vi "mpu.vi"() -> ()   [LabVIEW 2019]
panel:
  out "error out":errorcluster
  in  "error in":errorcluster {"code" format="%.0x"}
  in  "?":i32(slide)=7 scale=20.0..50.0
  in  "Вкл.":bool
  out "Крен, град":dbl(graph)
  out "Тангаж":cluster{i32, dbl}(graph)
  out "?":dbl
  out "Крен, град":dbl(knob) scale=-180.0..180.0
  out "?":dbl
  out "Тангаж, град.":dbl(knob) scale=-180.0..180.0
  in  "Порт:":refnum<visa-resource-name>
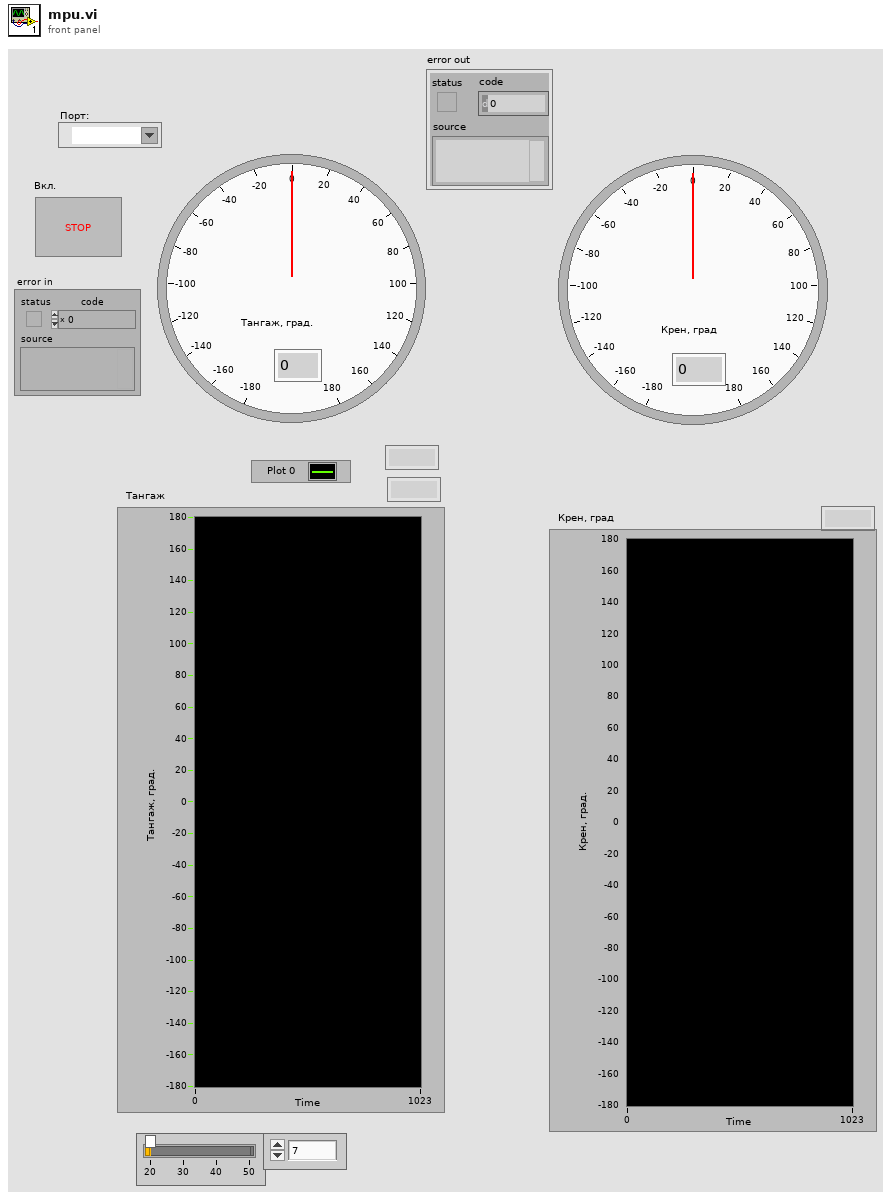
[diagram p1: front panel]
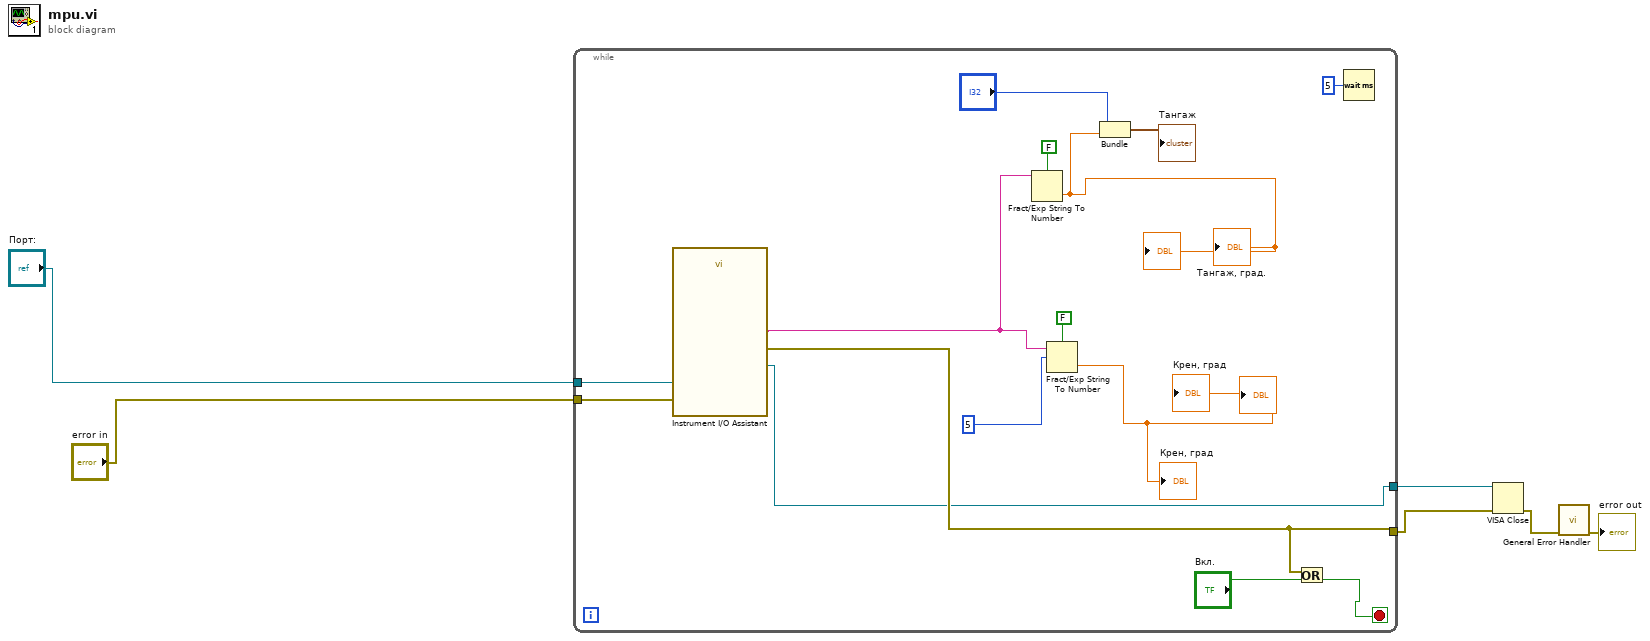
[diagram p0: block diagram]
diagram:
  n1 = while {
    tunnel: [w8] -> w6
    tunnel: "Порт:" -> [w11]
    tunnel: "error in" -> [w10]
    tunnel: [w7] -> w1
    stop <- w12 stop-if-true
    n2 = call "Instrument I/O Assistant"("Session In"=w11, "error in"=w10) -> ("Session Out"=w7:refnum<visa-resource-name>, "token"=w9:string, "error out"=w8:errorcluster)  [unwired: 23 in]
    n3 = Fract/Exp String To Number(use system decimal point (T)=FALSE, string=w9) -> (number=w16:dbl)  [unwired: 2 in, 1 out]
    "Тангаж, град." <- w16
    "?" <- w16
    n4 = Fract/Exp String To Number(use system decimal point (T)=FALSE, string=w9, offset=5) -> (number=→"Крен, град" →"?" →"Крен, град":dbl)  [unwired: 1 in, 1 out]
    n5 = Bundle("?", w16) -> (→"Тангаж":cluster{i32, dbl})  [unwired: 1 in]
    n6 = Or(x=w8, y="Вкл.") -> (x .or. y?=w12:bool)
    n7 = Wait (ms)(milliseconds to wait=u32 5) -> ()  [unwired: 1 out]
  }
  n8 = VISA Close(VISA resource name=w1, error in (no error)=w6) -> (error out=w5:errorcluster)
  n9 = call <vilib>:"General Error Handler.vi"("error in (no error)"=w5) -> ("error out"=→"error out":errorcluster)  [unwired: 10 in, 4 out]
